vi "LXM32_Read.vi"(6 "Timeout":u32=5000, 8 "error in":errorcluster, 9 "register param":T1, 10 "Slave Address":u8, 11 "VISA resource name":refnum<visa-resource-name>) -> (0 "error out":errorcluster, 2 "value":dbl, 3 "VISA resource name out":refnum<visa-resource-name>)   [LabVIEW 2015, in "LXM32_Modbus_Serial.lvlib"]
uses:
  LXM32_Modbus_Serial.lvlib
  register_param.ctl
  NI Modbus.llb/MB Serial Master Query Read Input Registers (poly).vi
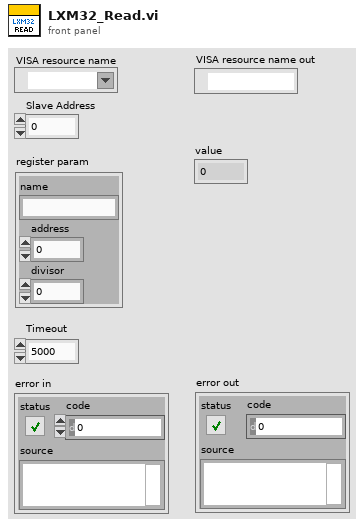
[diagram p1: front panel]
types:
  T1 = typedef "LXM32_Modbus_Serial.lvlib/register_param.ctl" = cluster{"name":string, "address":u16, "divisor":dbl}
  T2 = cluster{"Mode":enum16{"RTU", "ASCII"}, "Slave Address":u8}
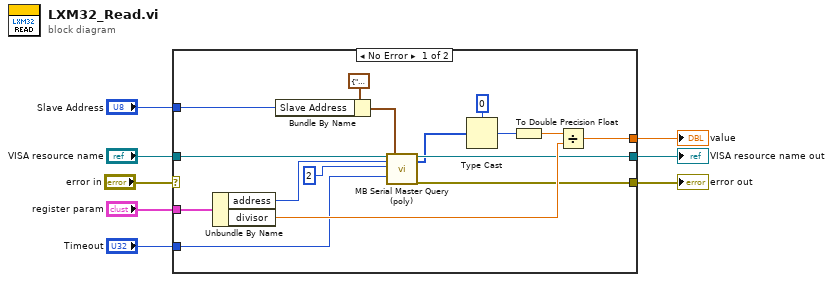
[diagram p0: block diagram]
diagram:
  n1 = case shown="No Error" "error in" {
    selector: "error in" -> [_ w25]
    tunnel: "VISA resource name" -> [w15 w26]
    tunnel: "register param" -> [w24 _]
    tunnel: "Timeout" -> [w12 _]
    tunnel: "Slave Address" -> [w22 _]
    tunnel: [w9 w25] -> w3
    tunnel: [w16 w26] -> w1
    tunnel: [w17 _] -> w2
    frame No Error {
      n2 = Unbundle By Name(w24) -> ("address"=w13:u16, "divisor"=w18:dbl)
      n3 = Bundle By Name(cluster=T2 {"Mode"=enum."RTU", "Slave Address"=0} ("Serial Parameters"), "Slave Address"=w22) -> (w11:T2)
      n4 = call-poly "MB Serial Master Query (poly).vi"("VISA resource name"=w15, "Starting Address"=w13, "Quantity"=u16 2, "Timeout"=w12, "Serial Parameters"=w11) -> ("VISA resource name out"=w16:refnum<visa-resource-name>, "Input Registers"=w10:u16[], "error out"=w9:errorcluster)  [unwired: 11 in, 1 out]
      n5 = Type Cast(type=0, x=w10) -> (*(type *) &x=w20:i32)
      n6 = To Double Precision Float(number=w20) -> (double precision float=w19:dbl)
      n7 = Divide(x=w19, y=w18) -> (x/y=w17:dbl)
    }
    frame Error {
    }
  }
  "error out" <- w3
  "VISA resource name out" <- w1
  "value" <- w2
